vi "Digital Pattern Gen 1.3 Validate Fault Positions.vi"(9 "max angle":dbl, 10 "end angle":dbl, 11 "start angle":dbl) -> (3 "valid":bool)   [LabVIEW 2019, in "Engine Simulation Toolkit Engine.lvlib"]
uses:
  Engine Simulation Toolkit Engine.lvlib
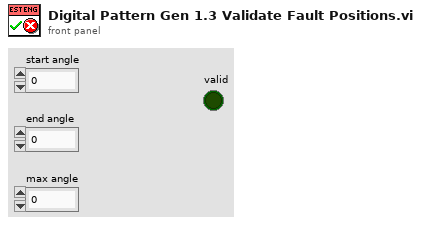
[diagram p1: front panel]
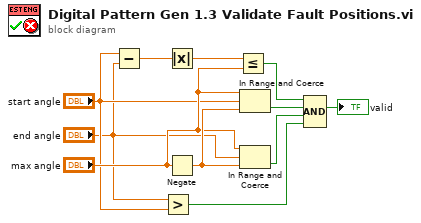
[diagram p0: block diagram]
diagram:
  n1 = Subtract(x="start angle", y="end angle") -> (x-y=w11:dbl)
  n2 = Greater?(x="end angle", y="start angle") -> (0:w1:bool)
  n3 = Absolute Value(x=w11) -> (abs(x)=w10:dbl)
  n4 = Negate(x="max angle") -> (-x=w9:dbl)
  n5 = Less Or Equal?(x=w10, y="max angle") -> (x <= y?=w7:bool)
  n6 = In Range and Coerce(upper limit="max angle", x="start angle", lower limit=w9) -> (In Range?=w6:bool)  [unwired: 1 out]
  n7 = In Range and Coerce(upper limit="max angle", x="end angle", lower limit=w9) -> (In Range?=w5:bool)  [unwired: 1 out]
  n8 = Compound Arithmetic op=AND(w7, w6, w5, w1) -> (→"valid":bool)
